vi "Display_Module.vi"(3 "Manual Controls.PSOCT Channel":u32, 4 "Acquisition mode":T1, 5 "Imaging Parameter.Line Averages":u8, 6 "Y":i32=1, 7 "X":i32=2048, 8 "error in":errorcluster, 9 "Z":i32=500, 10 "Source in":T2, 11 "Angle (degrees)":sgl) -> (0 "error out":errorcluster, 2 "AIP":T2(plugin-control) caption="Image")   [LabVIEW 2018]
uses:
  <vilib>/vision/Image Controls.llb/IMAQ Image.ctl
  type defines/FFT mode.ctl
  Controls/Queue Manager Actions.ctl
  <vilib>/vision/NI_Vision_Development_Module.lvlib
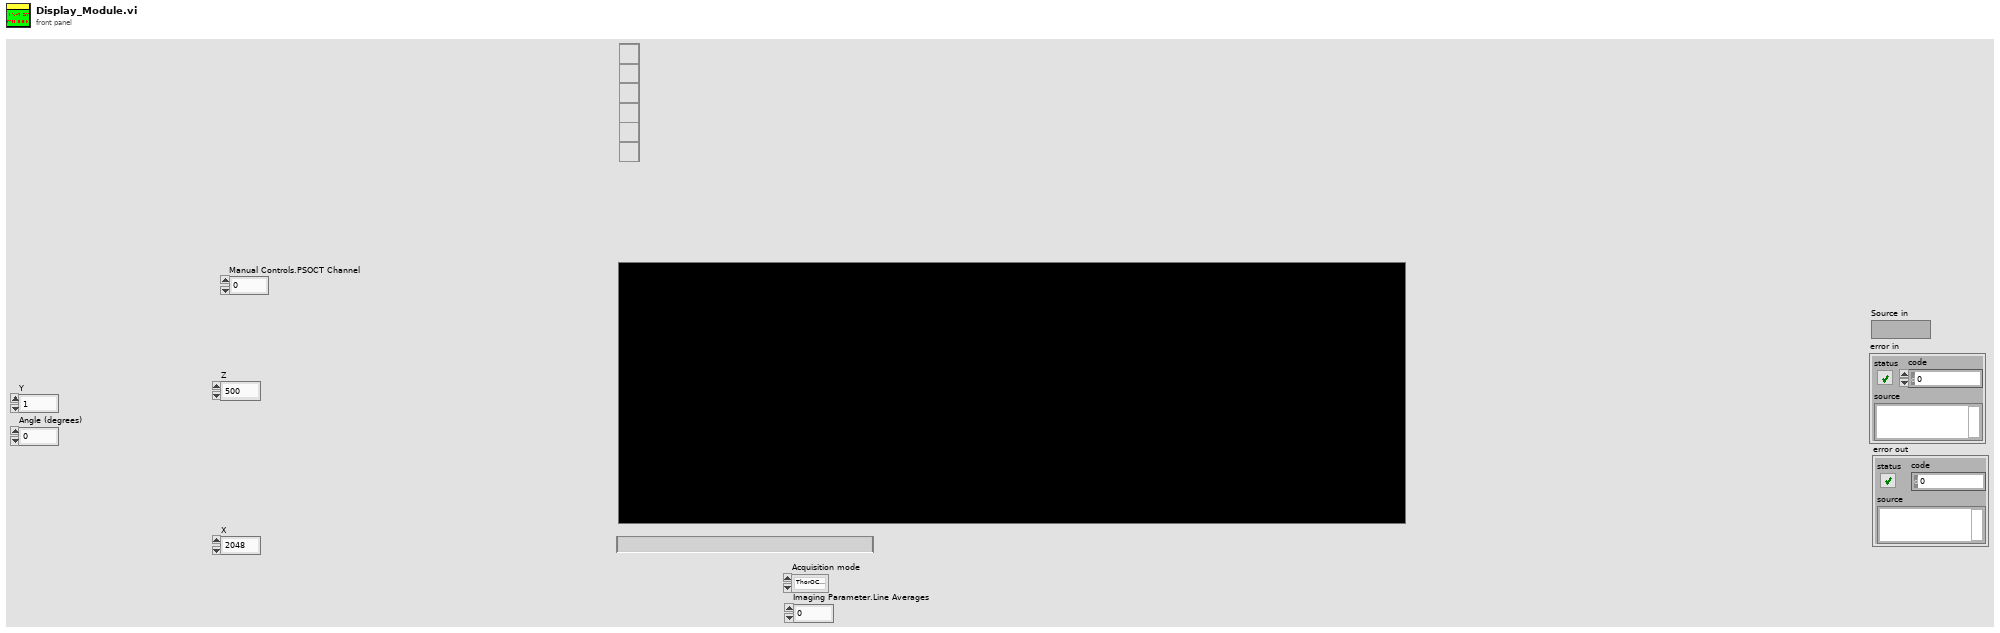
[diagram p1: front panel]
types:
  T1 = typedef "FFT mode.ctl" = enum16{"ThorOCT B line", "ThorOCT Spectral", "ThorOCT FFT", "Alazar B line", "Alazar FFT", "GPU FFT", "Alazar Spectral"}
  T2 = typedef "IMAQ Image.ctl" = refnum<image>
  T3 = typedef "Queue Manager Actions.ctl" = enum16{"Init", "Enqueue", "Enqueue All", "Preview Queue", "Dequeue", "Get Status", "Flush Queue", "Flush All Queues", "Release All Queues", "Release Queue", "Enqueue at Opposite End"}
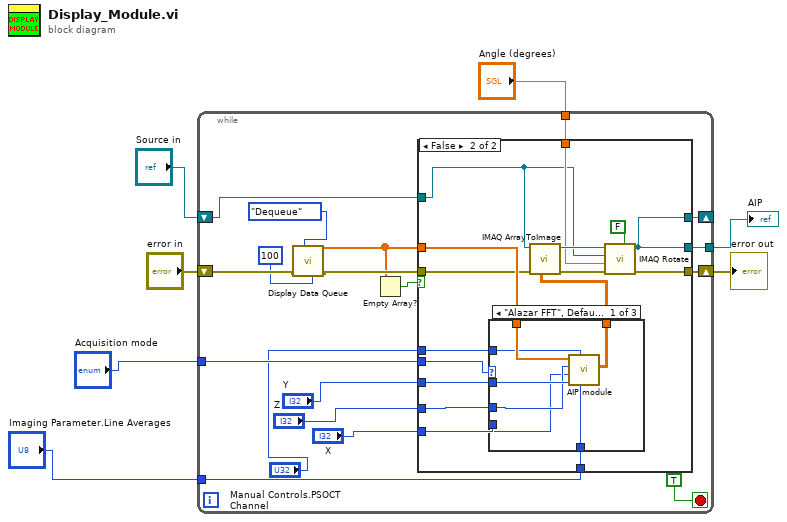
[diagram p0: block diagram]
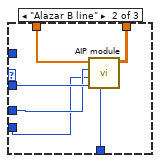
[diagram p3: hidden frame]
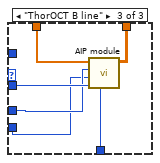
[diagram p4: hidden frame]
diagram:
  n1 = while {
    shift-right: [w25] -> w6
    shift-left: "error in" -> [w19]
    shift-right: [w22] -> _
    shift-left: "Source in" -> [w20]
    tunnel: [w21] -> w5
    tunnel: "Angle (degrees)" -> [w14]
    tunnel: "Acquisition mode" -> [w13]
    tunnel: "Imaging Parameter.Line Averages" -> [w9]
    stop <- TRUE stop-if-true
    n2 = call "Display Data Queue.vi"("timeout in ms (-1)"=100 ("time out"), "Action"=Queue_Manager_Actions."Dequeue", "error in (no error)"=w19) -> ("error out"=w18:errorcluster, "data out"=w17:sgl[])  [unwired: 5 in, 2 out]
    n3 = Empty Array?(array=w17) -> (empty?=w23:bool)
    n4 = case shown="False" w23 {
      tunnel: w18 -> [w27 w31]
      tunnel: [w27 w43] -> w25
      tunnel: w17 -> [_ w38]
      tunnel: [w26 w39] -> w22
      tunnel: [w26 w39] -> w21
      tunnel: w20 -> [w26 w30]
      tunnel: w14 -> [_ w37]
      tunnel: w13 -> [_ w29]
      tunnel: "Y" -> [_ w35]
      tunnel: "Z" -> [_ w34]
      tunnel: "X" -> [_ w33]
      tunnel: w9 -> [_ w32]
      tunnel: "Manual Controls.PSOCT Channel" -> [_ w28]
      frame True {
      }
      frame False {
        n5 = case shown="\"Alazar FFT\", Default" w29 {
          tunnel: w38 -> [w50 w56 w62]
          tunnel: [w49 w51 w57] -> w36
          tunnel: w35 -> [w48 w55 w61]
          tunnel: w34 -> [w47 w54 w60]
          tunnel: w33 -> [w46 w53 w59]
          tunnel: w32 -> [w45 w52 w58]
          tunnel: w28 -> [w44 _ _]
          frame "Alazar FFT", Default {
            n6 = call "AIP module.vi"("Imaging Parameter.Line Averages"=w45, "Manual Controls.PSOCT Channel"=w44, "Y"=w48, "X"=w46, "Z"=w47, "3D volume"=w50) -> ("AIP"=w49:sgl[][])  [unwired: 4 in, 1 out]
          }
          frame "Alazar B line" {
            n7 = call "AIP module.vi"("Imaging Parameter.Line Averages"=w52, "Y"=w55, "X"=w53, "Z"=w54, "3D volume"=w56) -> ("Bline"=w51:dbl[][])  [unwired: 5 in, 1 out]
          }
          frame "ThorOCT B line" {
            n8 = call "AIP module.vi"("Imaging Parameter.Line Averages"=w58, "Y"=w61, "X"=w59, "Z"=w60, "3D volume"=w62) -> ("Bline"=w57:dbl[][])  [unwired: 5 in, 1 out]
          }
        }
        n9 = call "IMAQ ArrayToImage"("Image Pixels (Float)"=w36, "error in (no error)"=w31, "Image"=w30) -> ("error out"=w41:errorcluster, "Image Out"=w42:T2)  [unwired: 7 in]
        n10 = call "IMAQ Rotate"("Maintain Size"=FALSE, "error in (no error)"=w41, "Angle (degrees)"=w37, "Image Dst"=w30, "Image Src"=w42) -> ("error out"=w43:errorcluster, "Image Dst Out"=w39:T2)  [unwired: 5 in]
      }
    }
  }
  "error out" <- w6
  "AIP" <- w5
